vi "setUp.vi"(8 "error in (no error)":errorcluster, 11 "Unit Tests for Runner in":refnum<class "Unit Tests for Runner.lvclass">) -> (0 "error out":errorcluster, 3 "Unit Tests for Runner out":refnum<class "Unit Tests for Runner.lvclass">)   [LabVIEW 2013, in "Unit Tests for Runner.lvclass"]
uses:
  Unit Tests for Runner.lvclass
  Unit Tests for Runner.lvclass/Unit Tests for Runner.ctl
  classes/Test Runner/Test Runner.lvclass
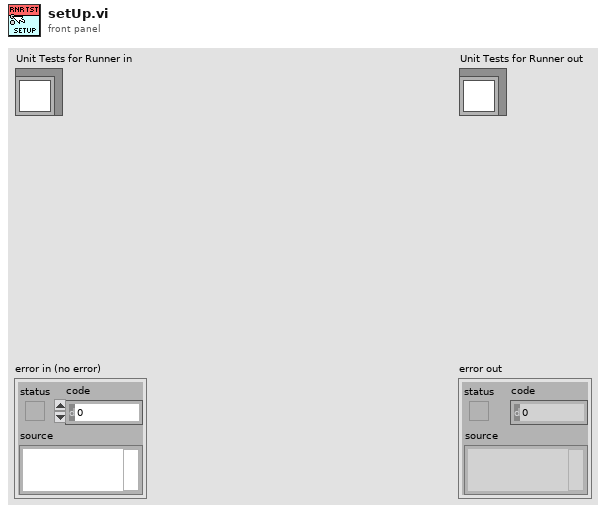
[diagram p1: front panel]
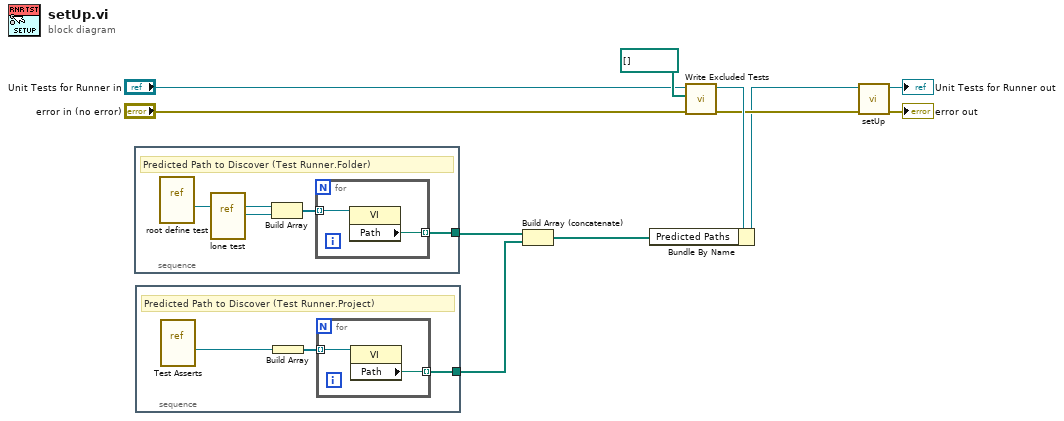
[diagram p0: block diagram]
diagram:
  n1 = stacked-sequence {
    tunnel: [w12] -> w6
    frame #0 {
      # "Predicted Path to Discover (Test Runner.Folder)"
      n2 = vi-ref "root define test.vi"() -> (w15:refnum<vi>)
      n3 = vi-ref "lone test.vi"() -> (w14:refnum<vi>)
      n4 = Build Array(w15, w14) -> (w13:refnum<vi>[])
      n5 = for {
        tunnel: w13 -> [w17] mode=indexing
        tunnel: [w16] -> w12 mode=indexing
        n6 = property on="Property Node" class="VI"(reference=w17) -> ("Path"=w16:path)  [unwired: 1 in, 2 out]
      }
    }
  }
  n7 = stacked-sequence {
    tunnel: [w18] -> w5
    frame #0 {
      # "Predicted Path to Discover (Test Runner.Project)"
      n8 = vi-ref "Test Asserts.vi"() -> (w20:refnum<vi>)
      n9 = Build Array(w20) -> (w19:refnum<vi>[])
      n10 = for {
        tunnel: w19 -> [w22] mode=indexing
        tunnel: [w21] -> w18 mode=indexing
        n11 = property on="Property Node" class="VI"(reference=w22) -> ("Path"=w21:path)  [unwired: 1 in, 2 out]
      }
    }
  }
  n12 = Build Array (concatenate)(w6, w5) -> (w4:path[])
  n13 = call "Write Excluded Tests.vi"("error in (no error)"="error in (no error)", "Excluded Tests"=path[] [], "Test Runner in"="Unit Tests for Runner in") -> ("error out"=w3:errorcluster, "Test Runner out"=w8:refnum<class "Unit Tests for Runner.lvclass">)  [unwired: 7 in]
  n14 = Bundle By Name(cluster=w8, "Predicted Paths"=w4) -> (w2:refnum<class "Unit Tests for Runner.lvclass">)
  n15 = call-parent "setUp.vi"("error in (no error)"=w3, "Test Runner in"=w2) -> ("error out"=→"error out":errorcluster, "Test Runner out"=→"Unit Tests for Runner out":refnum<class "Unit Tests for Runner.lvclass">)  [unwired: 8 in]
